vi "read maps.vi"(8 "error in":errorcluster, 10 "Data Form":T1, 11 "data value reference In":refnum<data-value>) -> (0 "error out":errorcluster, 2 "All Spectra":cluster{"Ramp Pattern":dbl[], "Array":i32[]}[](array[cluster]), 3 "data value reference out":refnum<data-value>)   [LabVIEW 2023]
uses:
  control/Data Form.ctl
  control/file structure.ctl
  <vilib>/Analysis/1siggen.llb/Ramp Pattern by Samples.vi
  <vilib>/Analysis/NI_AALBase.lvlib
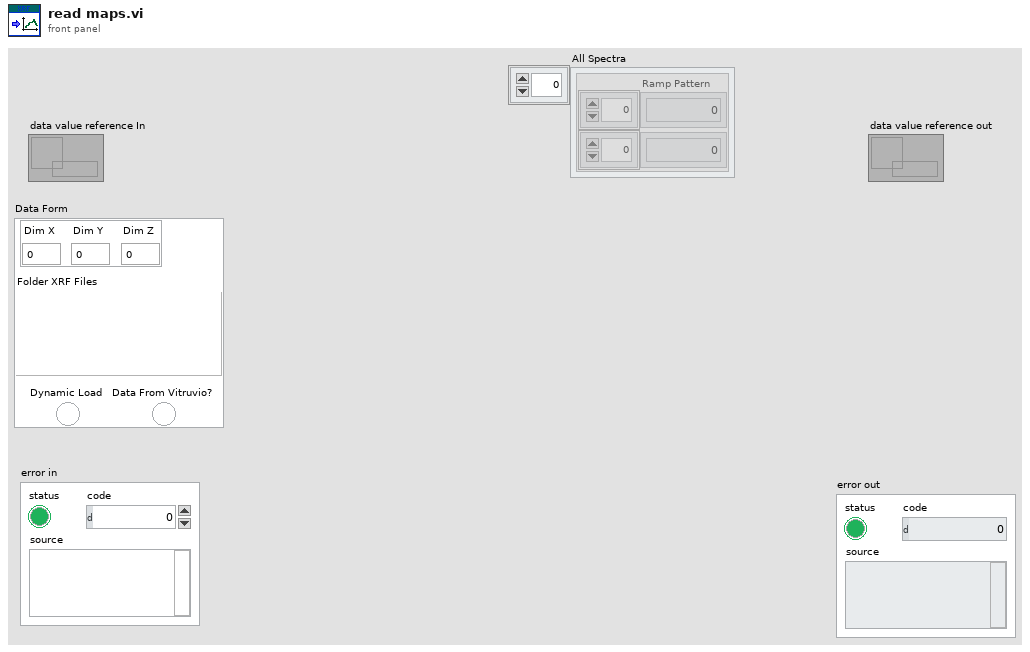
[diagram p1: front panel]
types:
  T1 = typedef "Data Form.ctl" = cluster{"Dimensions":cluster{"Dim X":i32, "Dim Y":i32, "Dim Z":i32}, "Folder XRF Files":path, "Dynamic Load":bool, "Data From Vitruvio?":bool}
  T2 = typedef "file structure.ctl" = cluster{"Colonna":i32, "Offset Righe":i32, "Coda Righe":i32, "Transpose":bool}
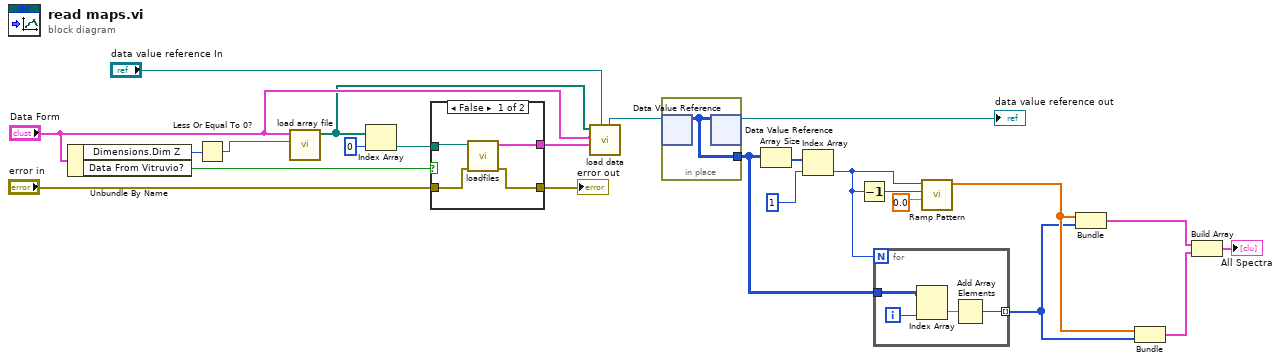
[diagram p0: block diagram]
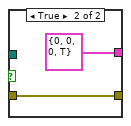
[diagram p2: hidden frame]
diagram:
  n1 = Unbundle By Name("Data Form") -> ("Dimensions.Dim Z"=w24:i32, "Data From Vitruvio?"=w21:bool)
  n2 = Less Or Equal To 0?(x=w24) -> (x <= 0?=w23:bool)
  n3 = call "load array file.vi"("2d?"=w23, "Data Form"="Data Form") -> ("File Array Out"=w16:path[])  [unwired: 9 in]
  n4 = Index Array(array=w16, index=0) -> (element=w20:path)
  n5 = case shown="False" w21 {
    tunnel: w20 -> [w28 _]
    tunnel: "error in" -> [w27 w30]
    tunnel: [w26 w30] -> w6
    tunnel: [w25 T2 {"Colonna"=0, "Offset Righe"=0, "Coda Righe"=0, "Transpose"=TRUE} ("File Structure")] -> w18
    frame False {
      n6 = call "loadfiles.vi"("Error In"=w27, "First Spectrum"=w28) -> ("Error Out"=w26:errorcluster, "File Structure"=w25:T2)  [unwired: 8 in]
    }
    frame True {
    }
  }
  "error out" <- w6
  n7 = call "load data.vi"("Data loaded reference In"="data value reference In", "File Structure"=w18, "Data Form"="Data Form", "File Array In"=w16) -> ("Data loaded reference Out"=w15:refnum<data-value>)  [unwired: 7 in]
  n8 = in-place {
    in-place-border: [w31] -> w7
    n9 = in-place-dvr #1(w15) -> (w31:i32[][])  [unwired: 1 out]
    n10 = in-place-dvr #1(w31) -> (→"data value reference out":refnum<data-value>)  [unwired: 1 out]
  }
  n11 = Array Size(array=w7) -> (size(s)=w11:i32[])
  n12 = Index Array(array=w11, index=1) -> (element=w8:i32)
  n13 = Decrement(x=w8) -> (x-1=w9:i32)
  n14 = for {
    N: w8 -> [_]
    tunnel: w7 -> [w34]
    tunnel: [w32] -> w1 mode=indexing
    i -> [w33]
    n15 = Index Array(array=w34, index (col)=w33) -> (element=w35:i32[])  [unwired: 1 in]
    n16 = Add Array Elements(numeric array=w35) -> (sum=w32:i32)
  }
  n17 = call-poly <vilib>:"Ramp Pattern.vi"("start"=0.0, "end"=w9, "samples"=w8) -> ("Ramp Pattern"=w2:dbl[])  [unwired: 7 in, 1 out]
  n18 = Bundle("Ramp Pattern"=w2, w1) -> (w4:cluster{"Ramp Pattern":dbl[], i32[]})  [unwired: 1 in]
  n19 = Bundle("Ramp Pattern"=w2, w1) -> (w5:cluster{"Ramp Pattern":dbl[], i32[]})  [unwired: 1 in]
  n20 = Build Array(w4, w5) -> (→"All Spectra":cluster{"Ramp Pattern":dbl[], i32[]}[])
